vi "MoveToPosition2.vi"(7 "In Contact in":bool, 10 "Position in":bool, 11 "UiDefinition 2":T1) -> (3 "In Contact out":bool)   [LabVIEW 2020]
uses:
  UIReferences.ctl
  D:/LabviewDXFViewer/LabviewDXFViewer/bin/Release/LabviewDXFViewer.exe
  LabviewDXFViewer/bin/Release/LabviewDXFViewer.exe
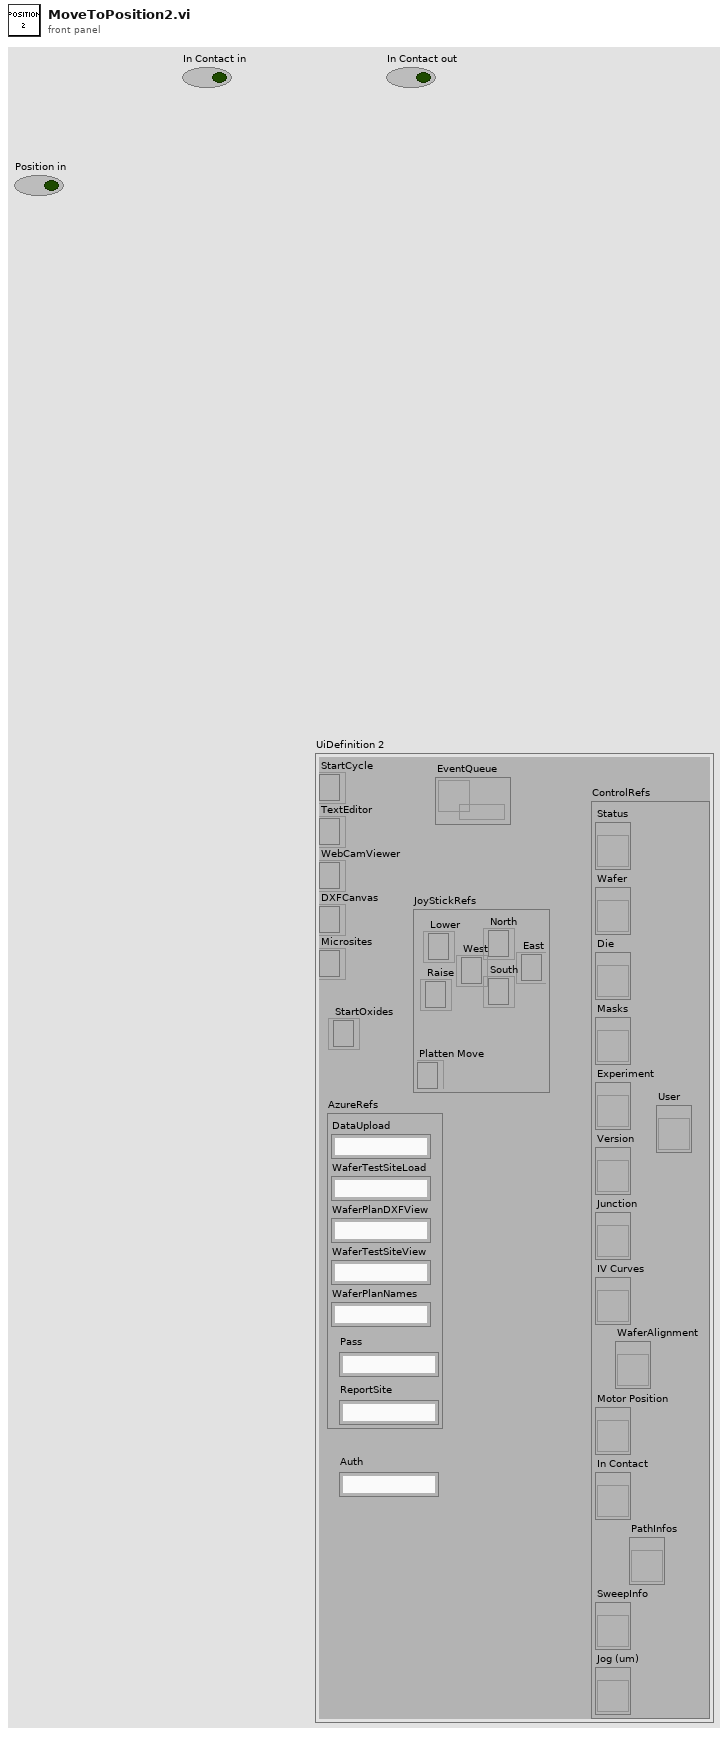
[diagram p1: front panel]
types:
  T1 = typedef "UIReferences.ctl" = cluster{"StartCycle":refnum<k24>, "TextEditor":refnum<k24>, "WebCamViewer":refnum<k24>, "DXFCanvas":refnum<k24>, "Microsites":refnum<k24>, "JoyStickRefs":cluster{"North":refnum<k24>, "Lower":refnum<k24>, "Raise":refnum<k24>, "Platten Move":refnum<k24>, "West":refnum<k24>, "East":refnum<k24>, "South":refnum<k24>}, "AzureRefs":cluster{"DataUpload":string, "WaferTestSiteLoad":string, "WaferPlanDXFView":string, "WaferTestSiteView":string, "WaferPlanNames":string, "Pass":string, "ReportSite":string}, "ControlRefs":cluster{"Status":refnum<vi>, "Wafer":refnum<vi>, "Die":refnum<vi>, "Masks":refnum<vi>, "Experiment":refnum<vi>, "Version":refnum<vi>, "Junction":refnum<vi>, "IV Curves":refnum<vi>, "Motor Position":refnum<vi>, "In Contact":refnum<vi>, "SweepInfo":refnum<vi>, "Jog (um)":refnum<vi>, "PathInfos":refnum<vi>, "User":refnum<vi>, "WaferAlignment":refnum<vi>}, "EventQueue":refnum<queue>, "StartOxides":refnum<k24>, "Auth":string}
  T2 = typedef "WaferAlignmentType.ctl" = cluster{"Wafer Units to microns":dbl, "Rotation Misalign":dbl[], "Scale Misalign":dbl, "Steps Per micron":dbl, "Position 1":i32[], "Position 2":i32[], "Lift Distance":i32, "Position 3":i32[], "Jog Height":i32}
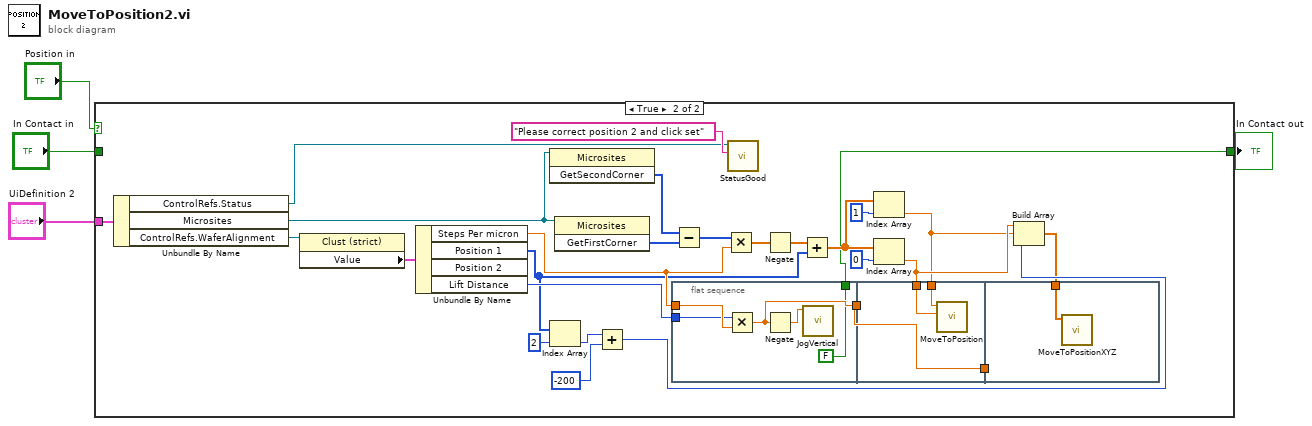
[diagram p0: block diagram]
diagram:
  n1 = case shown="True" "Position in" {
    tunnel: [w5 w19] -> w3
    tunnel: "In Contact in" -> [w5 _]
    tunnel: "UiDefinition 2" -> [_ w17]
    frame False {
    }
    frame True {
      n2 = Unbundle By Name(w17) -> ("ControlRefs.Status"=w15:refnum<vi>, "Microsites"=w14:refnum<k24>, "ControlRefs.WaferAlignment"=w18:refnum<vi>)
      n3 = property class="Clust (strict)"(reference=w18) -> ("Value"=w16:T2)  [unwired: 1 in, 2 out]
      n4 = Unbundle By Name(w16) -> ("Steps Per micron"=w21:dbl, "Position 1"=w11:i32[], "Lift Distance"=w20:i32)  [unwired: 1 out]
      n5 = invoke class="Microsites" method="GetSecondCorner"(reference=w14) -> ("GetSecondCorner"=w32:i32[])  [unwired: 2 in, 2 out]
      n6 = Index Array(array=w11, index=2) -> (element=w9:i32)
      n7 = invoke class="Microsites" method="GetFirstCorner"(reference=w14) -> ("GetFirstCorner"=w30:i32[])  [unwired: 2 in, 2 out]
      n8 = Add(x=w9, y=-200) -> (x+y=w7:i32)
      n9 = flat-sequence {
        tunnel: w21 -> [w36]
        tunnel: [w35] -> w27
        tunnel: w20 -> [w34]
        tunnel: [FALSE ("In Contact")] -> w19
        tunnel: w13 -> [w40]
        tunnel: w12 -> [w39]
        tunnel: [w38] -> w28
        tunnel: w27 -> [w38]
        tunnel: w28 -> [_]
        tunnel: w6 -> [w41]
        frame #0 {
          n10 = Multiply(x=w34, y=w36) -> (x*y=w35:dbl)
          n11 = Negate(x=w35) -> (-x=w37:dbl)
          n12 = call "JogVertical.vi"("Numeric"=w37) -> ()  [unwired: 11 in]
        }
        frame #1 {
          n13 = call "MoveToPosition.vi"("Y"=w40, "X"=w39) -> ()  [unwired: 10 in]
        }
        frame #2 {
          n14 = call "MoveToPositionXYZ.vi"("Array"=w41) -> ()  [unwired: 11 in]
        }
      }
      n15 = Subtract(x=w32, y=w30) -> (x-y=w31:i32[])
      n16 = Multiply(x=w31, y=w21) -> (x*y=w29:dbl[])
      n17 = call "StatusGood.vi"("Text.Text"="Please correct position 2 and click set" ("Status"), "String in"=w15) -> ()  [unwired: 10 in]
      n18 = Negate(x=w29) -> (-x=w23:dbl[])
      n19 = Add(x=w23, y=w11) -> (x+y=w24:dbl[])
      n20 = Index Array(array=w24, index=1) -> (element=w12:dbl)
      n21 = Index Array(array=w24, index=0) -> (element=w13:dbl)
      n22 = Build Array(w13, w12, w7) -> (w6:dbl[])
    }
  }
  "In Contact out" <- w3
